vi "Derivativo (SubVI).vi"(1 "Stop":bool, 2 "Kd":dbl, 3 "T":dbl, 4 "Vm":dbl) -> (0 "Accion Derivativa":dbl)   [LabVIEW 2011]
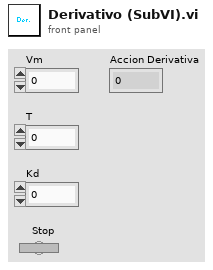
[diagram p1: front panel]
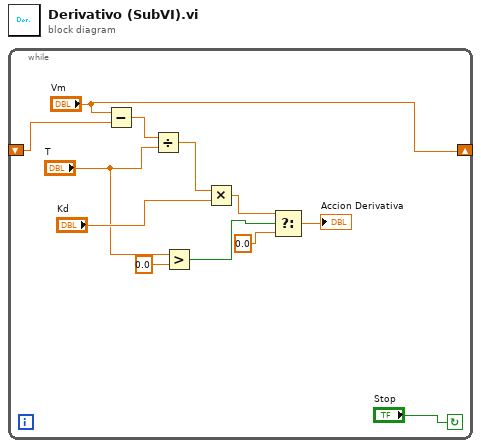
[diagram p0: block diagram]
diagram:
  n1 = while {
    shift-right: ["Vm"] -> _
    shift-left: _ -> [w3]
    stop <- "Stop" continue-if-true
    n2 = Subtract(x="Vm", y=w3) -> (x-y=w12:dbl)
    n3 = Divide(x=w12, y="T") -> (x/y=w11:dbl)
    n4 = Greater?(x="T", y=0.0) -> (0:w6:bool)
    n5 = Multiply(x=w11, y="Kd") -> (x*y=w7:dbl)
    n6 = Select(t=w7, s=w6, f=0.0) -> (s? t:f=→"Accion Derivativa":dbl)
  }
